vi "FTW-SyncServer-Construct.vi"(5 "Instance Inbox Address":string, 7 "Linger":i32=200 format="%d msec", 9 "Receive Message Size Limit":i32=1000000 format="%_4pbytes", 11 "error in":errorcluster) -> (4 "FTW Synchronous Server":refnum<data-value>, 6 "Resolved Inbox Address":string, 15 "error out":errorcluster)   [LabVIEW 2014]
doc: "Performs a \"cold call\" to connect to a running Actor Instance at the given Instance Inbox Address. Normally, this method is wrapped by a \"Construct\" method in each specific Actor Connector subclass."
uses:
  core/FTW-SyncServer-Core-Type.ctl
  error/FTW-ERR-ThrowGenericError.vi
  error/FTW-ERR-ThrowError.vi
  error/FTW-ERR-NoErrorConstant.vi
  error/FTW-ERR-CallChain.vi
  string/FTW-STR-ReplaceWhitespace.vi
panel:
  # "Inputs"
  # "Outputs"
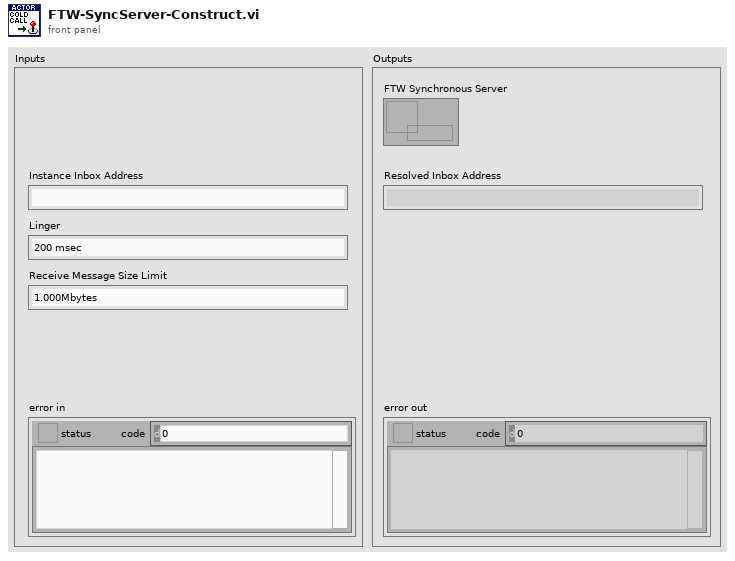
[diagram p1: front panel]
types:
  T1 = typedef "FTW-SyncServer-Core-Type.ctl" = cluster{"Socket":i64}
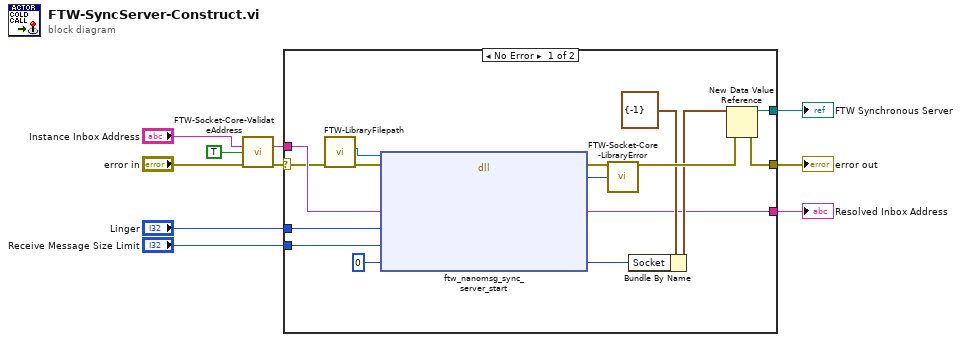
[diagram p0: block diagram]
diagram:
  n1 = call "FTW-Socket-Core-ValidateAddress.vi"("Address"="Instance Inbox Address", "Allow wildcard replacement?"=TRUE, "error in"="error in") -> ("Sanitized Address"=w5:string, "error out"=w6:errorcluster)  [unwired: 10 in, 1 out]
  n2 = case shown="No Error" w6 {
    selector: w6 -> [w17 w27]
    tunnel: [w24 w27] -> w10
    tunnel: w5 -> [w19 _]
    tunnel: [w23 _] -> w9
    tunnel: "Receive Message Size Limit" -> [w15 _]
    tunnel: "Linger" -> [w14 _]
    tunnel: [w11 _] -> w1
    frame No Error {
      n3 = call "FTW-LibraryFilepath.vi"("error in"=w17) -> ("error out"=w20:errorcluster, "Library Filepath"=w22:path)  [unwired: 8 in, 1 out]
      n4 = dll-call lib="?" fn="ftw_nanomsg_sync_server_start"(path in=w22, error in=w20, "Remote Address"=w19, "Linger (msec)"=w14, "Max Recv Size (bytes)"=w15, "Socket Handle"=i64 0) -> (error out=w21:errorcluster, "Return Value"=w16:i64, "Remote Address"=w11:string, "Socket Handle"=w12:i64)  [unwired: 5 in, 1 out]
      n5 = call "FTW-Socket-Core-LibraryError.vi"("error in"=w21, "Return Value"=w16) -> ("error out"=w26:errorcluster)  [unwired: 13 in]
      n6 = Bundle By Name(cluster=T1 {"Socket"=-1} ("FTW Synchronous Server"), "Socket"=w12) -> (w13:T1)
      n7 = New Data Value Reference(data value=w13, error in=w26) -> (data value reference=w23:refnum<data-value>, error out=w24:errorcluster)
    }
    frame Error {
    }
  }
  "error out" <- w10
  "FTW Synchronous Server" <- w9
  "Resolved Inbox Address" <- w1
